vi "ZMC Execute Get Remain Buff Space.vi"(8 "error in (no error)":errorcluster caption="错误输入（无错误）", 11 "handle":u32) -> (0 "error out":errorcluster caption="错误输出", 2 "function return":u32, 3 "handle out":u32)   [LabVIEW 2015, in "zauxdll.lvlib"]
doc: "uint32 __stdcall ZMC_ExecuteGetRemainBuffSpace(ZMC_HANDLE handle);"
uses:
  zauxdll.lvlib
  zmotion.dll
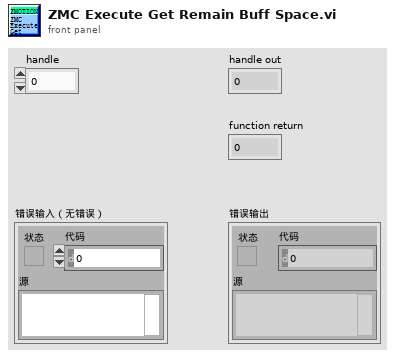
[diagram p1: front panel]
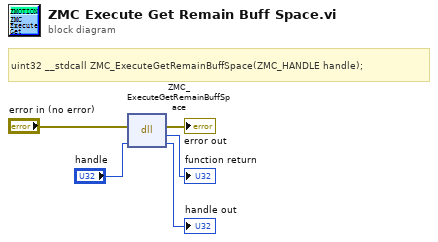
[diagram p0: block diagram]
diagram:
  # "uint32 __stdcall ZMC_ExecuteGetRemainBuffSpace(ZMC_HANDLE handle);"
  n1 = dll-call lib="C:/Users/VIC/Desktop/GOGORO_SA/system/LLB/zmotion/zaux/zmotion.*" fn="ZMC_ExecuteGetRemainBuffSpace"(error in="error in (no error)", "handle"="handle") -> (error out=→"error out":errorcluster, →"function return":u32, "handle"=→"handle out":u32)  [unwired: 2 in, 1 out]
